vi "Run all tests CLI.vi"   [LabVIEW 2020]
uses:
  <vilib>/addons/_JKI Toolkits/Caraya/classes/Test Report/Test Report.lvclass
  <vilib>/addons/_JKI Toolkits/Caraya/classes/Test Suite/Test Suite.lvclass
  <vilib>/Wiresmith Technology/G CLI/CLI Class/CLI.lvclass
  <vilib>/addons/_JKI Toolkits/Caraya/classes/Test Result/Test Result.lvclass
  <vilib>/addons/_JKI Toolkits/Caraya/Caraya.lvlib
  <vilib>/addons/_JKI Toolkits/Caraya/run-tests/Run Test (Scalar Path).vi
types:
  T1 = enum32{"Invalid", "Standard", "Closed", "Hidden", "Minimized", "Maximized"}
  T2 = typedef "Caraya.lvlib/Test Result.lvclass/Node Results (Extended).ctl" = cluster{"Test Node":T3, "Assertions":T5[]}
  T3 = typedef "Caraya.lvlib/Test Result.lvclass/Test Node (Extended).ctl" = cluster{"Test Registration":T4, "Defined":bool, "Passed":bool, "properties":variant}
  T4 = typedef "Caraya.lvlib/Test Result.lvclass/Test Registration Data.ctl" = cluster{"Name":string, "Call Chain":string[], "Time Stamp":timestamp, "Test ID":string, "Caller ID":string}
  T5 = typedef "Caraya.lvlib/Test Result.lvclass/Assert Event Data (Extended).ctl" = cluster{"name":string, "passed":bool, "call-chain":string[], "test-error":errorcluster, "timestamp":timestamp, "assert-id":string, "test-id":string, "time":dbl, "message":string, "properties":variant, "measurements":variant, "user-defined":variant}
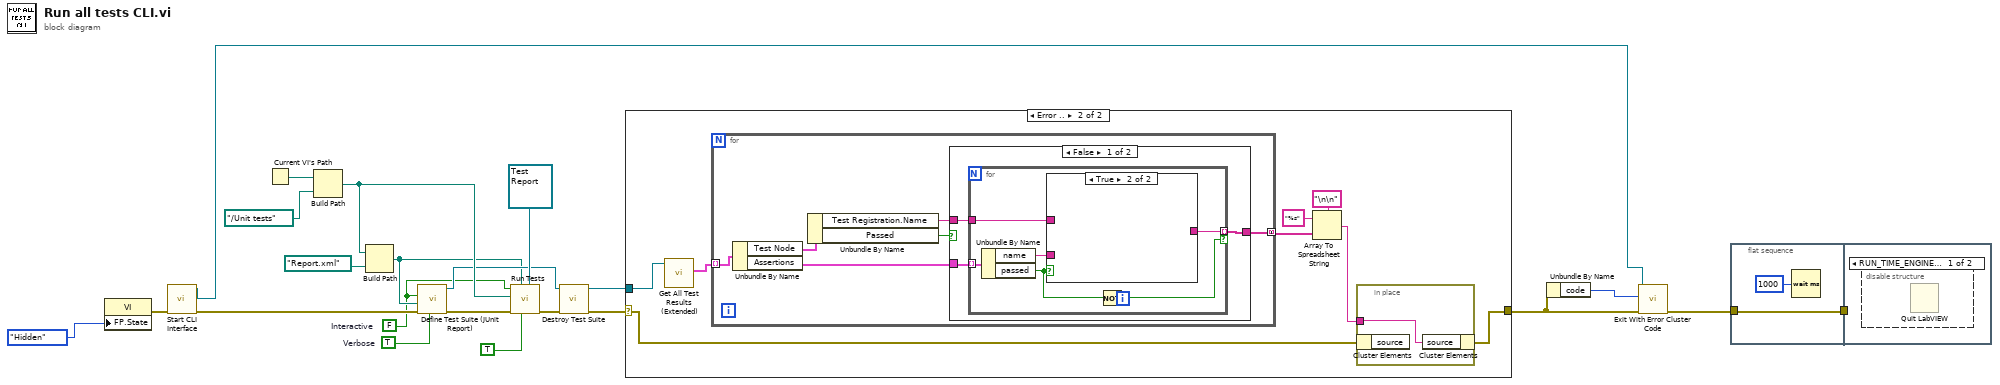
[diagram p0: block diagram]
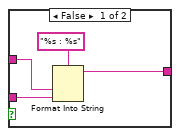
[diagram p4: hidden frame]
diagram:
  w14 = TRUE  # Verbose
  w3 = FALSE  # Interactive
  n1 = property class="VI"("FP.State"=T1."Hidden" ("Front Panel Window:State")) -> (error out=w10:errorcluster)  [unwired: 2 in, 1 out]
  n2 = call <vilib>:"Start CLI Interface.vi"("error in (no error)"=w10) -> ("error out"=w5:errorcluster, "CLI out"=w8:refnum<class "CLI.lvclass">)  [unwired: 7 in, 2 out]
  n3 = Current VI's Path() -> (path=w21:path)
  n4 = Build Path(base path=w21, name or relative path=path "../Unit tests") -> (appended path=w18:path)
  n5 = Build Path(base path=w18, name or relative path=path "Report.xml") -> (appended path=w13:path)
  n6 = call <vilib>:"Define Test Suite (JUnit Report).vi"("Verbose (F)"=w14, "error in (no error)"=w5, "Report Path"=w13, "Interactive"=w3) -> ("error out"=w12:errorcluster, "Test Suite"=w15:refnum<class "Test Suite.lvclass">)  [unwired: 5 in, 1 out]
  n7 = call-poly <vilib>:"Run Tests.vi"("Test Report"=refnum<class "Test Report.lvclass"> refnum, "Verbose"=TRUE, "Report Path"=w13, "error in"=w12, "Test Path"=w18, "Interactive (T)"=w3) -> ("error out"=w11:errorcluster)  [unwired: 4 in, 1 out]
  n8 = call-dynamic "Destroy Test Suite.vi"("error in (no error)"=w11, "Test Suite in"=w15) -> ("error out"=w7:errorcluster, "Test Suite Results"=w16:refnum<class "Test Result.lvclass">)  [unwired: 8 in]
  n9 = case shown="Error .." w7 {
    selector: w7 -> [w23 w26]
    tunnel: w16 -> [_ w31]
    tunnel: [w23 w24] -> w6
    frame No Error {
    }
    frame Error {
      n10 = call <vilib>:"Get All Test Results (Extended).vi"("Test Result in"=w31) -> ("Test Results"=w27:T2[])  [unwired: 8 in, 2 out]
      n11 = for {
        tunnel: w27 -> [w37] mode=indexing
        tunnel: [w33] -> w28 mode=concatenating
        n12 = Unbundle By Name(w37) -> ("Test Node"=w36:T3, "Assertions"=w38:T5[])
        n13 = Unbundle By Name(w36) -> ("Test Registration.Name"=w34:string, "Passed"=w35:bool)
        n14 = case shown="False" w35 {
          tunnel: w38 -> [w41 _]
          tunnel: w34 -> [w40 _]
          tunnel: [w39 _] -> w33
          frame False {
            n15 = for {
              tunnel: w41 -> [w47] mode=indexing
              tunnel: w40 -> [w45]
              tunnel: [w44] -> w39 mode=indexing if=w42
              n16 = Unbundle By Name(w47) -> ("name"=w46:string, "passed"=w43:bool)
              n17 = case shown="True" w43 {
                tunnel: w46 -> [w50 _]
                tunnel: w45 -> [w51 _]
                tunnel: [w48 _] -> w44
                frame False {
                  n18 = Format Into String(format string="%s : %s", w51, w50) -> (resulting string=w48:string)  [unwired: 2 in, 1 out]
                }
                frame True {
                }
              }
              n19 = Not(x=w43) -> (.not. x?=w42:bool)
            }
          }
          frame True {
          }
        }
      }
      n20 = Array To Spreadsheet String(delimiter (Tab)="\n\n", array=w28, 3:"%s" ("format string")) -> (spreadsheet string=w25:string)
      n21 = in-place {
        in-place-border: w25 -> [w32]
        n22 = in-place-cluster #1(w26) -> ()  [unwired: 1 out]
        n23 = in-place-cluster #1("source"=w32) -> (w24:errorcluster)
      }
    }
  }
  n24 = Unbundle By Name(w6) -> ("code"=w22:i32)
  n25 = call <vilib>:"Exit With Error Cluster Code.vi"("error in (no error)"=w6, "No Error Code (0)"=w22, "CLI in"=w8) -> ("error out"=w1:errorcluster)  [unwired: 8 in]
  n26 = flat-sequence {
    tunnel: w1 -> [w53]
    tunnel: [w53] -> w2
    tunnel: w2 -> [_]
    frame #0 {
      n27 = Wait (ms)(milliseconds to wait=u32 1000) -> ()  [unwired: 1 out]
    }
    frame #1 {
      n28 = disable-structure shown="RUN_TIME_ENGINE==True" {
        frame condition #0 {
          n29 = Quit LabVIEW() -> ()  [unwired: 1 in]
        }
        frame condition #1 (active) {
        }
      }
    }
  }
